vi "#253_MAV_MSG_STATUSTEXT.vi"(11 "mavlink_payload":u8[](array[numeric])) -> (3 "STATUSTEXT":T1)   [LabVIEW 2023]
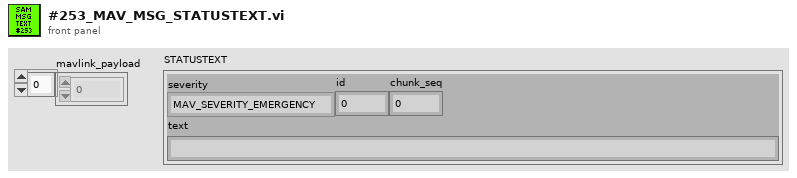
[diagram p1: front panel]
types:
  T1 = cluster{"severity":enum8{"MAV_SEVERITY_EMERGENCY", "MAV_SEVERITY_ALERT", "MAV_SEVERITY_CRITICAL", "MAV_SEVERITY_ERROR", "MAV_SEVERITY_WARNING", "MAV_SEVERITY_NOTICE", "MAV_SEVERITY_INFO", "MAV_SEVERITY_DEBUG"}, "id":u16, "chunk_seq":u8, "text":string}
  T2 = enum8{"MAV_SEVERITY_EMERGENCY", "MAV_SEVERITY_ALERT", "MAV_SEVERITY_CRITICAL", "MAV_SEVERITY_ERROR", "MAV_SEVERITY_WARNING", "MAV_SEVERITY_NOTICE", "MAV_SEVERITY_INFO", "MAV_SEVERITY_DEBUG"}
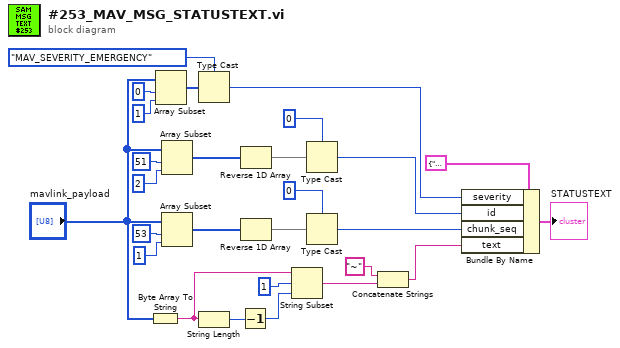
[diagram p0: block diagram]
diagram:
  n1 = Byte Array To String(unsigned byte array="mavlink_payload") -> (string=w24:string)
  n2 = Array Subset(array="mavlink_payload", index=0 ("Index"), length=1) -> (w16:u8[])
  n3 = Array Subset(array="mavlink_payload", index=51 ("Index"), length=2) -> (w11:u8[])
  n4 = Array Subset(array="mavlink_payload", index=53 ("Index"), length=1) -> (w5:u8[])
  n5 = Type Cast(type=T2."MAV_SEVERITY_EMERGENCY" ("severity"), x=w16) -> (*(type *) &x=w15:T2)
  n6 = String Length(string=w24) -> (length=w25:i32)
  n7 = Decrement(x=w25) -> (x-1=w26:i32)
  n8 = Reverse 1D Array(array=w11) -> (reversed array=w10:u8[])
  n9 = Reverse 1D Array(array=w5) -> (reversed array=w4:u8[])
  n10 = String Subset(string=w24, offset (0)=1, length (rest)=w26) -> (substring=w20:string)
  n11 = Type Cast(type=u16 0 ("Index"), x=w10) -> (*(type *) &x=w8:u16)
  n12 = Type Cast(type=u8 0 ("Index"), x=w4) -> (*(type *) &x=w1:u8)
  n13 = Concatenate Strings("~" ("string"), w20) -> (w19:string)
  n14 = Bundle By Name(cluster=T1 {"severity"=enum."MAV_SEVERITY_EMERGENCY", "id"=0, "chunk_seq"=0, "text"=""} ("STATUSTEXT"), "severity"=w15, "id"=w8, "chunk_seq"=w1, "text"=w19) -> (→"STATUSTEXT":T1)
